vi "DueDACtoAURORA.vi"() -> ()   [LabVIEW 2011]
uses:
  <vilib>/rvi/interface/RandomDataEmulation/nirviRandomDataFPGAFIFO.vi
  <vilib>/rvi/interface/RandomDataEmulation/niFpgaRandomDataHandleErrors.vi
  <vilib>/rvi/eio/common/nirviEmuTemplateMethod_errors.vi
  <vilib>/rvi/DataTransferAndStorage/Container/XNode/niFpgaContainer.xnode
  <vilib>/rvi/interface/RandomDataEmulation/nirviRandomDataFpgaReadWriteTemplate.vi
  <vilib>/eio/EIONode/EIONode.xnode
  <vilib>/rvi/Analysis/measure/butterworth/XNode/niFpgaButterworthFilter.xnode
  <vilib>/rvi/FXPMathLib/FxpAdd/XNode/nifxpmath_Add.xnode
  <vilib>/rvi/FXPMathLib/FxpMul/XNode/nifxpmath_Multiplier.xnode
  <vilib>/rvi/FXPMathLib/sim/FxpSim.dll
panel:
  out "length out reset":fxp<+/-,17,10>
  in  "Reset Mode":bool=TRUE
  in  "Lowpass filter\nForce":i16(ring)=2 items=["No Filter", "20 Hz", "60 Hz", "100 Hz"]
  out "filtered force":fxp<+/-,30,9>
  out "raw force":fxp<+/-,26,5>
  in  "length offset (V)":fxp<+/-,12,5>
  in  "Lowpass filter\nLength":i16(ring)=1 items=["No Filter", "60 Hz", "100 Hz"]
  in  "Gandalf volts/rad":fxp<+/-,17,6>=12.33984375
  in  "abs length limit (V)":fxp<+/-,12,5>=9.0
  out "offset dac":fxp<+/-,27,6>
  out "Mujoco\nmodel position\n(radians)":fxp<+/-,26,5>
  in  "DU dac gain":fxp<+/-,16,2>=1.25
  in  "DU dac\noffset":fxp<+/-,16,1>=-0.555999755859375
  out "from DUE dac0":fxp<+/-,26,5>
  out "loop time (ticks)":u32
  out "length out (V)":fxp<+/-,17,10>
  in  "Reset":bool=TRUE
  in  "Timeout":i32
  out "Full Flag\nTimed Out?":bool
  # "NOTE: Dac output has\nto be truncated so only\n2 digits of precision due\nto uncertainty of the rest."
  # "Gain and offset to compensate for limitations of Arduino DUE\nDAC"
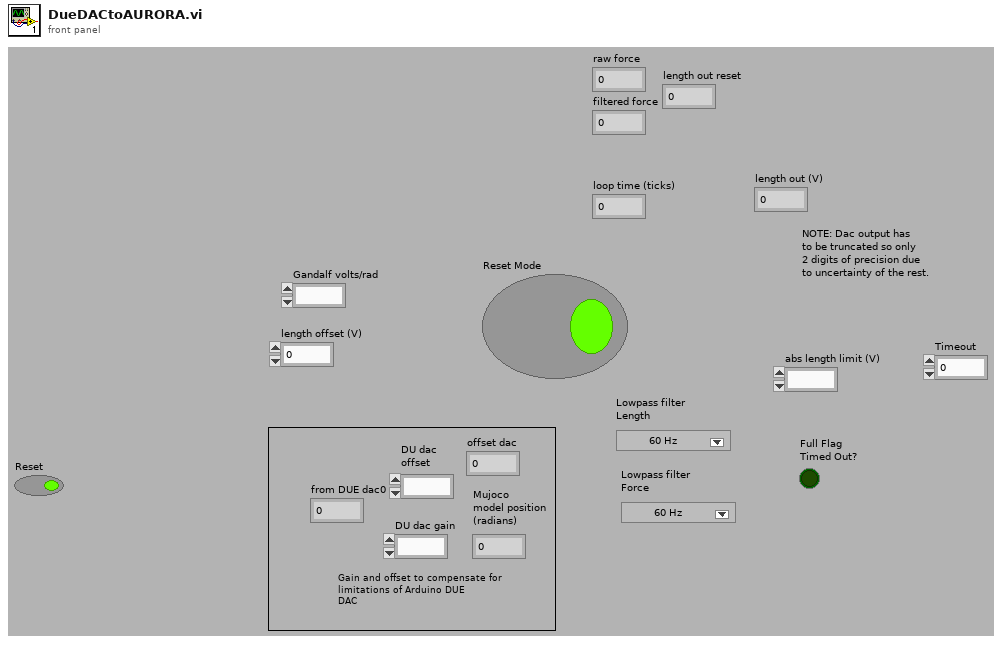
[diagram p1: front panel]
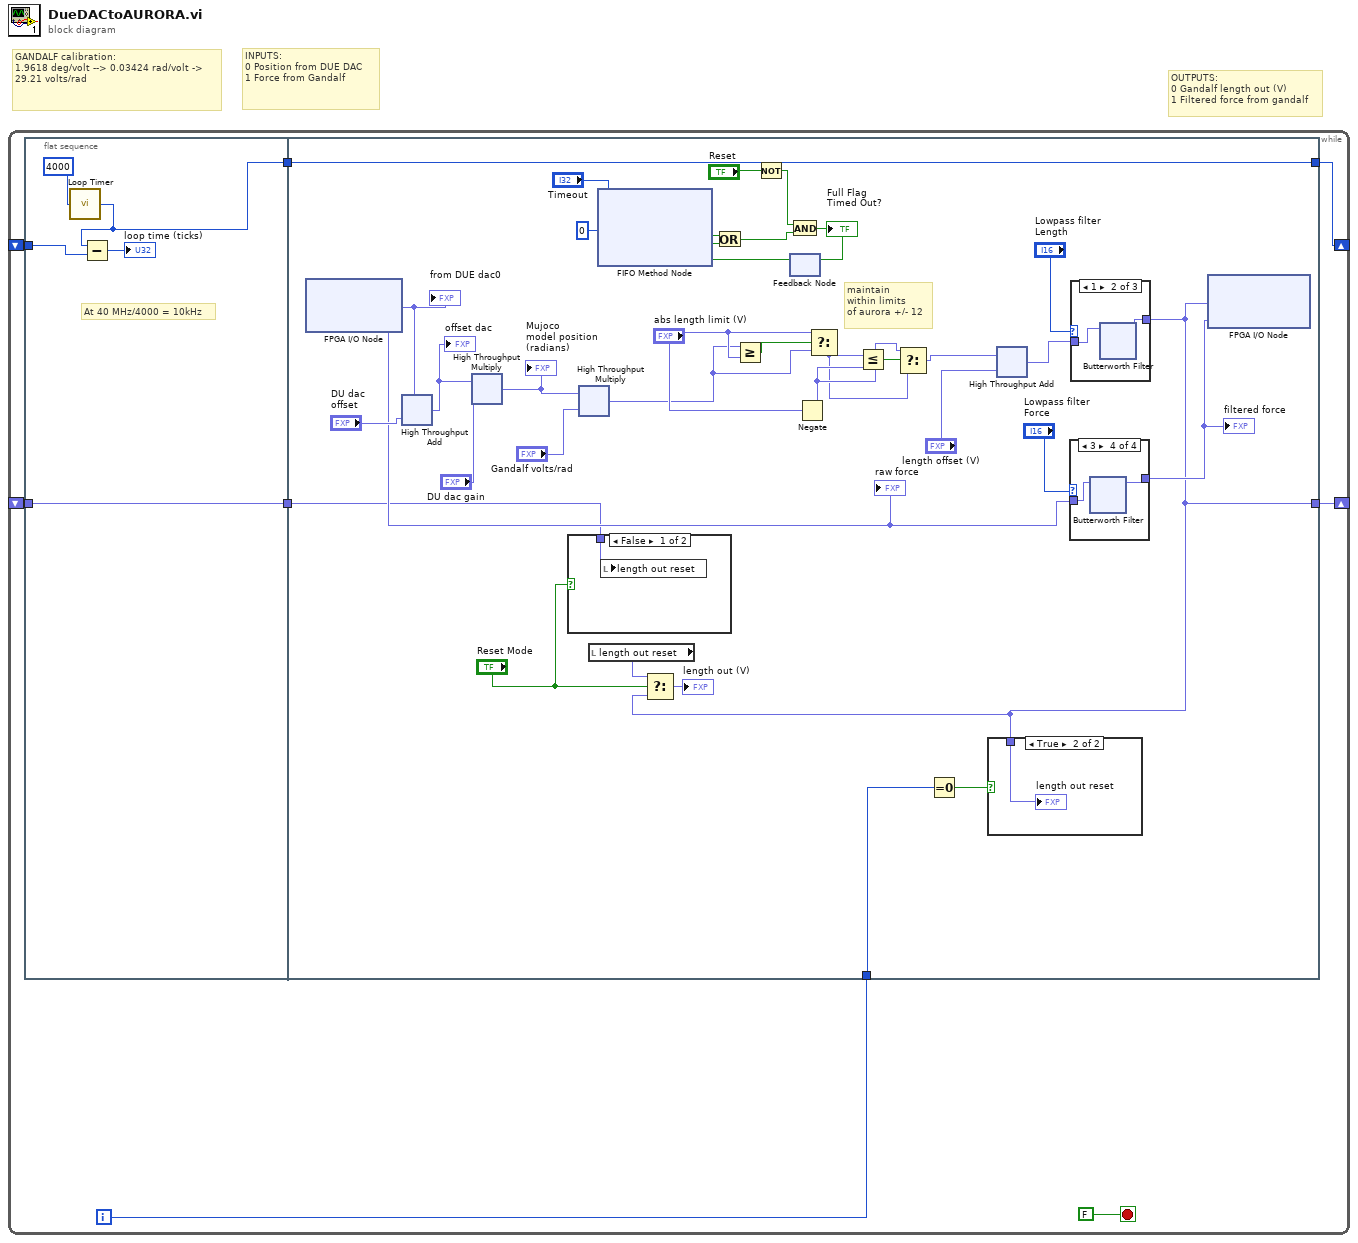
[diagram p0: block diagram]
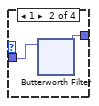
[diagram p5: hidden frame]
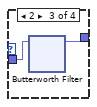
[diagram p6: hidden frame]
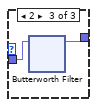
[diagram p8: hidden frame]
diagram:
  # "GANDALF calibration:\n1.9618 deg/volt --> 0.03424 rad/volt ->\n29.21 volts/rad"
  # "INPUTS:\n0 Position from DUE DAC\n1 Force from Gandalf"
  # "OUTPUTS:\n0 Gandalf length out (V)\n1 Filtered force from gandalf"
  n1 = while {
    shift-right: [w7] -> _
    shift-left: _ -> [w5]
    shift-right: [w4] -> _
    shift-left: _ -> [w2]
    i -> [w1]
    stop <- FALSE stop-if-true
    n2 = flat-sequence {
      tunnel: [w11] -> w6
      tunnel: w5 -> [w12]
      tunnel: [w9] -> w3
      tunnel: w2 -> [w9]
      tunnel: [w41] -> w7
      tunnel: w6 -> [w41]
      tunnel: [w15] -> w4
      tunnel: w3 -> [w20]
      tunnel: w1 -> [w16]
      frame #0 {
        # "At 40 MHz/4000 = 10kHz"
        n3 = call "Loop Timer"("Count(Ticks)"=u32 4000) -> ("Tick Count(Ticks)"=w11:u32)
        n4 = Subtract(x=w11, y=w12) -> (x-y=→"loop time (ticks)":u32)
      }
      frame #1 {
        # "maintain \nwithin limits\nof aurora +/- 12"
        n5 = xnode "FPGA I/O Node"() -> ("Mod2/AI0"=w31:fxp<+/-,26,5>, "Mod2/AI1"=w23:fxp<+/-,26,5>)  [unwired: 2 in, 2 out]
        "from DUE dac0" <- w31
        "raw force" <- w23
        n6 = xnode "High Throughput Add"("x"=w31, "y"="DU dac\noffset") -> ("x+y"=w32:fxp<+/-,26,5>)
        "offset dac" <- w32
        n7 = xnode "High Throughput Multiply"("x"=w32, "y"="DU dac gain") -> ("x*y"=w29:fxp<+/-,26,5>)
        "Mujoco\nmodel position\n(radians)" <- w29
        n8 = case shown="False" "Reset Mode" {
          tunnel: w20 -> [w50 _]
          frame False {
            n9 = local write "length out reset"(w50) -> ()
          }
          frame True {
          }
        }
        n10 = xnode "High Throughput Multiply"("x"=w29, "y"="Gandalf volts/rad") -> ("x*y"=w28:fxp<+/-,12,5>)
        n11 = local read "length out reset"() -> (w14:fxp<+/-,17,10>)
        n12 = xnode ("FIFO Method Node")("Element"=i16 0, "Timeout"="Timeout") -> ("Timed Out?"=w47:bool)  [unwired: 1 in, 1 out]
        n13 = Greater Or Equal?(x=w28, y="abs length limit (V)") -> (x >= y?=w39:bool)
        n14 = Not(x="Reset") -> (.not. x?=w45:bool)
        n15 = feedback #1() -> (w42:bool)  [unwired: 1 in]
        n16 = Or(x=w42, y=w47) -> (x .or. y?=w44:bool)
        n17 = And(x=w45, y=w44) -> (x .and. y?=w43:bool)
        "Full Flag\nTimed Out?" <- w43
        n18 = feedback-in #1(w43) -> ()
        n19 = Negate(x="abs length limit (V)") -> (-x=w36:fxp<+/-,13,6>)
        n20 = Select(t="abs length limit (V)", s=w39, f=w28) -> (s? t:f=w35:fxp<+/-,12,5>)
        n21 = Less Or Equal?(x=w35, y=w36) -> (x <= y?=w37:bool)
        n22 = Select(t=w36, s=w37, f=w35) -> (s? t:f=w25:fxp<+/-,13,6>)
        n23 = Equal To 0?(x=w16) -> (x = 0?=w17:bool)
        n24 = xnode "High Throughput Add"("x"=w25, "y"="length offset (V)") -> ("x+y"=w24:fxp<+/-,12,5>)
        n25 = case shown="3" "Lowpass filter\nForce" {
          tunnel: w23 -> [w51 w53 w62 w71]
          tunnel: [w51 w52 w61 w70] -> w22
          frame 0, Default {
          }
          frame 1 {
            n26 = xnode "Butterworth Filter"("input data"=w53) -> ("output data"=w52:fxp<+/-,30,9>)  [unwired: 2 in]
          }
          frame 2 {
            n27 = xnode "Butterworth Filter"("input data"=w62) -> ("output data"=w61:fxp<+/-,30,9>)  [unwired: 2 in]
          }
          frame 3 {
            n28 = xnode "Butterworth Filter"("input data"=w71) -> ("output data"=w70:fxp<+/-,30,9>)  [unwired: 2 in]
          }
        }
        "filtered force" <- w22
        n29 = case shown="1" "Lowpass filter\nLength" {
          tunnel: w24 -> [w80 w82 w91]
          tunnel: [w80 w81 w90] -> w15
          frame 0, Default {
          }
          frame 1 {
            n30 = xnode "Butterworth Filter"("input data"=w82) -> ("output data"=w81:fxp<+/-,16,9>)  [unwired: 2 in]
          }
          frame 2 {
            n31 = xnode "Butterworth Filter"("input data"=w91) -> ("output data"=w90:fxp<+/-,16,9>)  [unwired: 2 in]
          }
        }
        n32 = Select(t=w14, s="Reset Mode", f=w15) -> (s? t:f=→"length out (V)":fxp<+/-,17,10>)
        n33 = case shown="True" w17 {
          tunnel: w15 -> [_ w49]
          frame False {
          }
          frame True {
            "length out reset" <- w49
          }
        }
        n34 = xnode "FPGA I/O Node"("Mod1/AO0"=w15, "Mod1/AO1"=w22) -> ()  [unwired: 2 in, 2 out]
      }
    }
  }
